vi "Read Channel Info.vi"(8 "error in (no error)":errorcluster, 11 "Photon Counter SR400.lvclass in":refnum<class "Photon Counter SR400.lvclass">) -> (0 "error out":errorcluster, 1 "Channel Units":string[](array[string]), 2 "Channel Names":string[](array[string]), 3 "Photon Counter SR400.lvclass out":refnum<class "Photon Counter SR400.lvclass">, 5 "#Channels":i32)   [LabVIEW 2009, in "Photon Counter SR400.lvclass"]
doc: "(Dynamic) Return information about the readable data channels this object provides, e.g., the name of each data source and its unit."
uses:
  Photon Counter SR400.lvclass
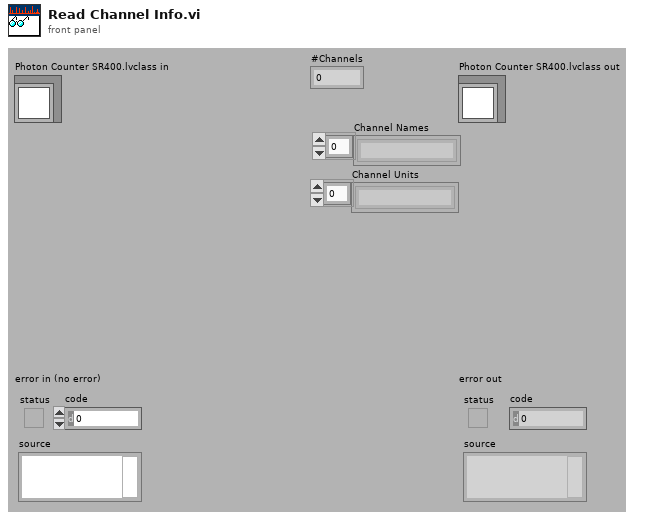
[diagram p1: front panel]
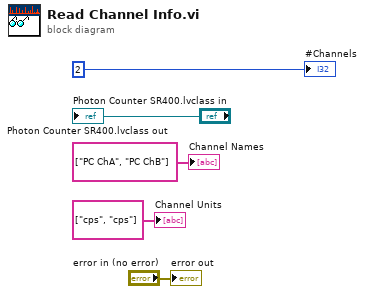
[diagram p0: block diagram]
diagram:
  "error out" <- "error in (no error)"
  "Photon Counter SR400.lvclass out" <- "Photon Counter SR400.lvclass in"
  "Channel Units" <- string[] ["cps", "cps"] ("Channel Units")
  "Channel Names" <- string[] ["PC ChA", "PC ChB"] ("Channel Names")
  "#Channels" <- 2 ("#Channels")
